vi "uploadfile.vi"(7 "error in (no error)":errorcluster, 8 "File Name on Drive":string, 9 "Local Path":path, 10 "Google Drive Service Ref":refnum<k24>) -> (0 "error out":errorcluster)   [LabVIEW 2016, in "GDrive.lvlib"]
doc: "This VI takes in a file path and a Google Drive Service Reference, and uploads the file at the path to the corresponding Google Drive."
uses:
  GDrive.lvlib
  C:/Users/motoole/Desktop/VC OToolekit/Dependencies/Google.Apis.Drive.v3.dll
  Dependencies/Google.Apis.Drive.v3.dll
  <vilib>/Utility/config.llb/Read Key (String).vi
  <vilib>/Utility/config.llb/NI_LVConfig.lvlib
panel:
  # "Provide the Google Drive Service Reference, the path of a \nlocal file, and the name of the file for the drive."
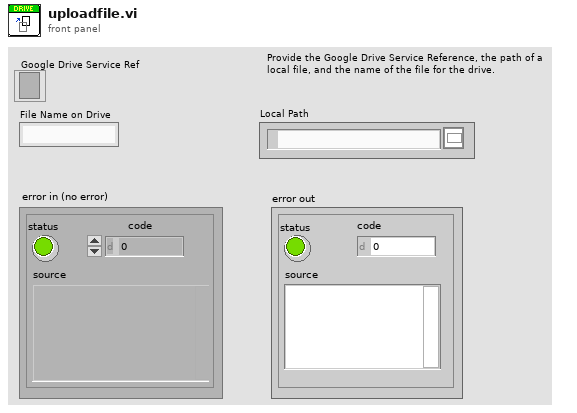
[diagram p1: front panel]
types:
  T1 = typedef "NI_LVConfig.lvlib/Config Data RefNum.ctl" = refnum<k1>
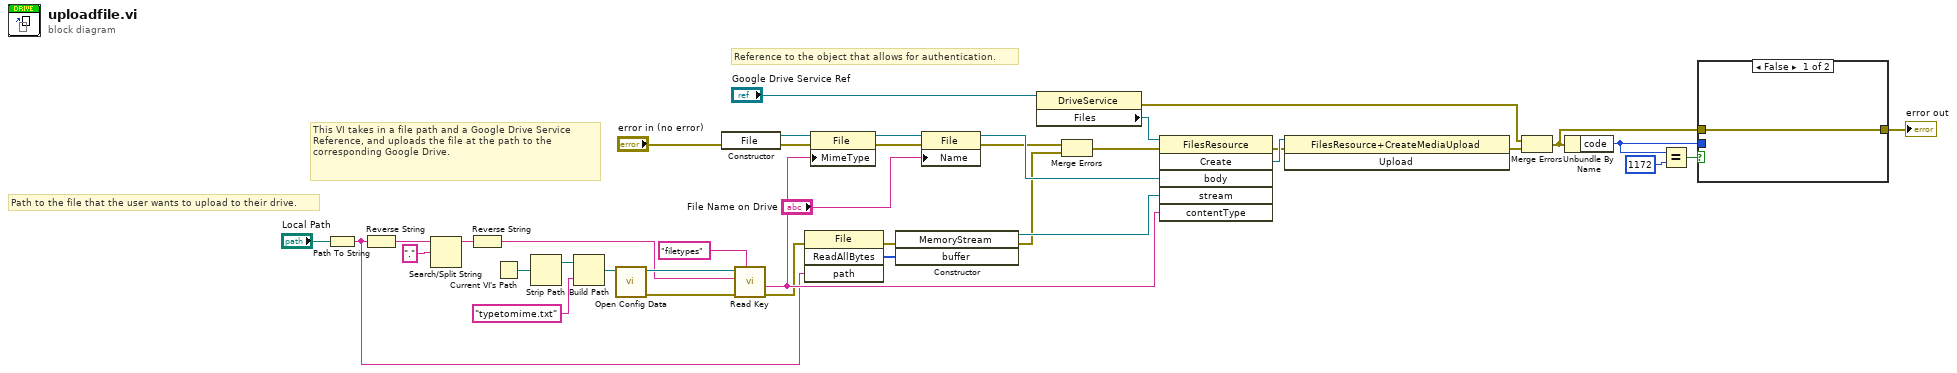
[diagram p0: block diagram]
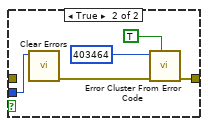
[diagram p2: hidden frame]
diagram:
  # "Path to the file that the user wants to upload to their drive."
  # "Reference to the object that allows for authentication."
  # "This VI takes in a file path and a Google Drive Service Reference, and uploads the file at the path to the corresponding Google Drive."
  n1 = Path To String(path="Local Path") -> (string=w6:string)
  n2 = Reverse String(1:w6) -> (0:w32:string)
  n3 = Search/Split String(string=w32, search string/char (-)=".") -> (substring before match=w33:string)  [unwired: 1 in, 2 out]
  n4 = Reverse String(1:w33) -> (0:w36:string)
  n5 = Current VI's Path() -> (path=w2:path)
  n6 = Strip Path(path=w2) -> (stripped path=w1:path)  [unwired: 1 out]
  n7 = Build Path(base path=w1, name or relative path="typetomime.txt") -> (appended path=w12:path)
  n8 = call <vilib>:"Open Config Data.vi"("configuration file path"=w12) -> ("error out"=w17:errorcluster, "refnum"=w37:T1)  [unwired: 8 in, 1 out]
  n9 = constructor class="File"(error in="error in (no error)") -> (reference out=w24:refnum<k24>, error out=w39:errorcluster)  [unwired: 2 in, 1 out]
  n10 = call-poly <vilib>:"Read Key.vi"("section"="filetypes", "error in (no error)"=w17, "key"=w36, "refnum"=w37) -> ("error out"=w18:errorcluster, "value"=w38:string)  [unwired: 4 in, 2 out]
  n11 = invoke class="File" method="ReadAllBytes"(error in=w18, "path"=w6) -> (error out=w19:errorcluster, "ReadAllBytes"=w25:u8[])  [unwired: 2 in, 2 out]
  n12 = property class="File"(reference=w24, error in=w39, "MimeType"=w38) -> (reference out=w29:refnum<k24>, error out=w21:errorcluster)
  n13 = constructor class="MemoryStream"(error in=w19, "buffer"=w25) -> (reference out=w26:refnum<k24>, error out=w15:errorcluster)  [unwired: 2 in, 2 out]
  n14 = property class="File"(reference=w29, error in=w21, "Name"="File Name on Drive") -> (reference out=w30:refnum<k24>, error out=w16:errorcluster)
  n15 = property class="DriveService"(reference="Google Drive Service Ref") -> (error out=w5:errorcluster, "Files"=w23:refnum<k24>)  [unwired: 1 in, 1 out]
  n16 = Merge Errors(w16, w15) -> (w14:errorcluster)
  n17 = invoke class="FilesResource" method="Create"(reference=w23, error in=w14, "body"=w30, "stream"=w26, "contentType"=w38) -> (error out=w20:errorcluster, "Create"=w27:refnum<k24>)  [unwired: 1 in, 4 out]
  n18 = invoke class="FilesResource+CreateMediaUpload" method="Upload"(reference=w27, error in=w20) -> (error out=w4:errorcluster)  [unwired: 1 in, 2 out]
  n19 = Merge Errors(w5, w4) -> (w3:errorcluster)
  n20 = Unbundle By Name(w3) -> ("code"=w8:i32)
  n21 = Equal?(x=w8, y=1172) -> (x = y?=w9:bool)
  n22 = case shown="False" w9 {
    tunnel: w8 -> [_ w45]
    tunnel: [w40 w43] -> w7
    tunnel: w3 -> [w40 _]
    frame False {
    }
    frame True {
      n23 = call <vilib>:"Clear Errors.vi"("specific error code to clear (0: all)"=w45) -> ("error out"=w44:errorcluster)  [unwired: 5 in, 1 out]
      n24 = call <vilib>:"Error Cluster From Error Code.vi"("show call chain? (False)"=TRUE, "error in (no error)"=w44, "error code (0)"=403464) -> ("error out"=w43:errorcluster)  [unwired: 6 in]
    }
  }
  "error out" <- w7
